vi "Initialize.vi"(8 "error in":errorcluster, 11 "ELAN data unit (ADU) in":refnum<class "ELAN Data Unit.lvclass">) -> (0 "error out":errorcluster, 3 "ELAN data unit (ADU) out":refnum<class "ELAN Data Unit.lvclass">)   [LabVIEW 2021, in "ELAN Data Unit.lvclass"]
doc: "This provides an interface for the master to open a connection to the slave."
uses:
  ELAN Data Unit.lvclass
  ELAN Data Unit.lvclass/ELAN Data Unit.ctl
  <vilib>/Instr/_visa.llb/VISA Flush IO Buffer Mask.ctl
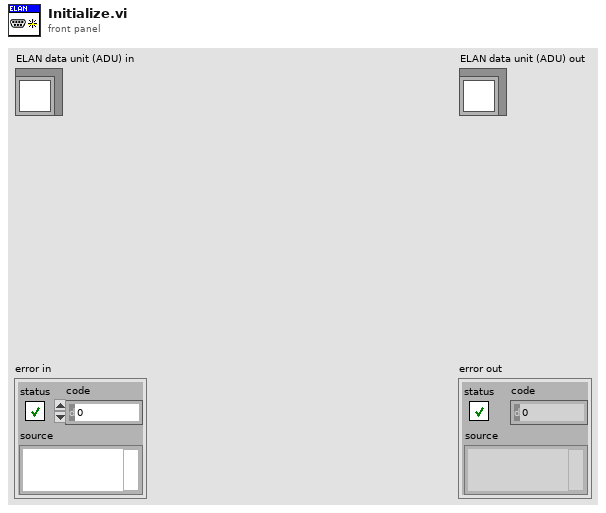
[diagram p1: front panel]
types:
  T1 = typedef "VISA Flush IO Buffer Mask.ctl" = u16
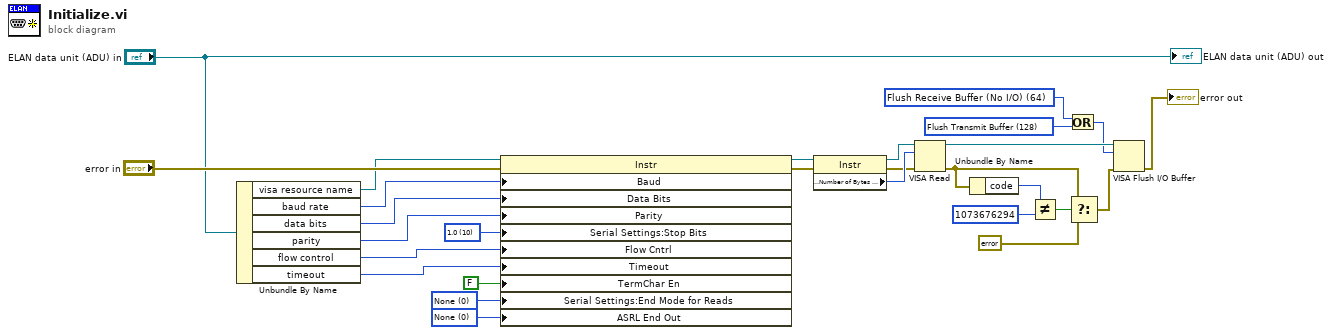
[diagram p0: block diagram]
diagram:
  w1 = u16 0 items=["None", "Last Bit", "TermChar", "Break"] ("Serial Settings:End Mode for Writes")
  w2 = u16 0 items=["None", "Last Bit", "TermChar"] ("Serial Settings:End Mode for Reads")
  w6 = u16 10 items=["1.0"=10, "1.5"=15, "2.0"=20] ("Serial Settings:Stop Bits")
  w23 = T1 128 items=["Flush Receive Buffer"=16, "Write Transmit Buffer to Device"=32, "Flush Receive Buffer (No I/O)"=64, "Flush Transmit Buffer"=128] ("Mask")
  w22 = T1 64 items=["Flush Receive Buffer"=16, "Write Transmit Buffer to Device"=32, "Flush Receive Buffer (No I/O)"=64, "Flush Transmit Buffer"=128] ("Mask")
  n1 = Unbundle By Name("ELAN data unit (ADU) in") -> ("visa resource name"=w10:refnum<visa-resource-name>, "baud rate"=w9:u32, "data bits"=w8:u16, "parity"=w7:u16, "flow control"=w5:u16, "timeout"=w3:u32)
  n2 = property class="Instr"(reference=w10, error in="error in", "Baud"=w9, "Data Bits"=w8, "Parity"=w7, "Serial Settings:Stop Bits"=w6, "Flow Cntrl"=w5, "Timeout"=w3, "TermChar En"=FALSE ("Message Based Settings:Termination Character Enable"), "Serial Settings:End Mode for Reads"=w2, "ASRL End Out"=w1) -> (reference out=w25:refnum<visa-resource-name>, error out=w24:errorcluster)
  n3 = property class="Instr"(reference=w25, error in=w24) -> (reference out=w27:refnum<visa-resource-name>, error out=w20:errorcluster, "Serial Settings:Number of Bytes at Serial Port"=w28:u32)
  n4 = VISA Read(VISA resource name=w27, byte count=w28, error in (no error)=w20) -> (VISA resource name out=w26:refnum<visa-resource-name>, error out=w15:errorcluster)  [unwired: 2 out]
  n5 = Unbundle By Name(w15) -> ("code"=w19:i32)
  n6 = Not Equal?(x=w19, y=1073676294) -> (x != y?=w17:bool)
  n7 = Or(x=w22, y=w23) -> (x .or. y?=w21:T1)
  n8 = Select(t=w15, s=w17, f=errorcluster {"status"=FALSE, "code"=0, "source"=""}) -> (s? t:f=w14:errorcluster)
  n9 = VISA Flush I/O Buffer(VISA resource name=w26, mask (16)=w21, error in (no error)=w14) -> (error out=→"error out":errorcluster)  [unwired: 1 out]
  "ELAN data unit (ADU) out" <- "ELAN data unit (ADU) in"
